vi "Menu-Stop Acq CNV.vi"(11 "Menu in":refnum<k9>) -> ()   [LabVIEW 2016, in "CML UI.lvlib"]
uses:
  CML UI.lvlib
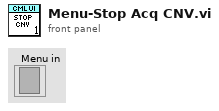
[diagram p1: front panel]
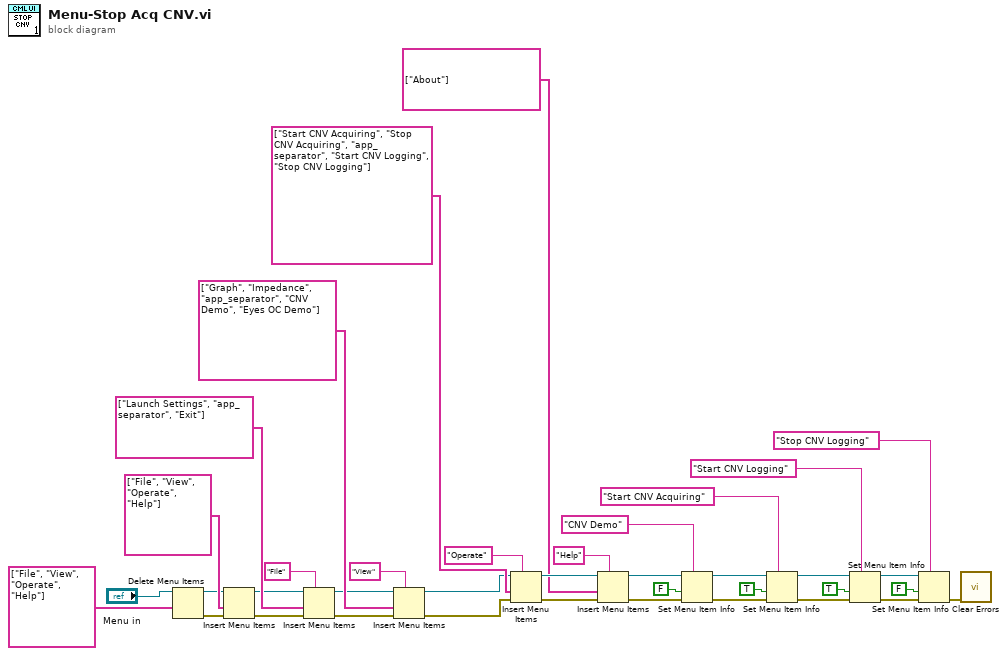
[diagram p0: block diagram]
diagram:
  n1 = Delete Menu Items(7:string[] ["File", "View", "Operate", "Help"] ("L10n_item tags 1"), 9:"Menu in") -> (0:w11:errorcluster, 3:w12:refnum<k9>)  [unwired: 2 in]
  n2 = Insert Menu Items(6:w11, 7:string[] ["File", "View", "Operate", "Help"] ("L10n_item tags 1"), 9:w12) -> (0:w27:errorcluster, 3:w25:refnum<k9>)  [unwired: 3 in, 1 out]
  n3 = Insert Menu Items(5:"File" ("L10n_menu tag"), 6:w27, 7:string[] ["Launch Settings", "app_separator", "Exit"] ("L10n_item tags 2"), 9:w25) -> (0:w32:errorcluster, 3:w31:refnum<k9>)  [unwired: 2 in, 1 out]
  n4 = Insert Menu Items(5:"View" ("L10n_menu tag"), 6:w32, 7:string[] ["Graph", "Impedance", "app_separator", "CNV Demo", "Eyes OC Demo"] ("L10n_item tags 2"), 9:w31) -> (0:w36:errorcluster, 3:w35:refnum<k9>)  [unwired: 2 in, 1 out]
  n5 = Insert Menu Items(5:"Operate" ("L10n_menu tag"), 6:w36, 7:string[] ["Start CNV Acquiring", "Stop CNV Acquiring", "app_separator", "Start CNV Logging", "Stop CNV Logging"] ("L10n_item tags 2"), 9:w35) -> (0:w22:errorcluster, 3:w23:refnum<k9>)  [unwired: 2 in, 1 out]
  n6 = Insert Menu Items(5:"Help" ("L10n_menu tag"), 6:w22, 7:string[] ["About"] ("L10n_item tags 2"), 9:w23) -> (0:w18:errorcluster, 3:w20:refnum<k9>)  [unwired: 2 in, 1 out]
  n7 = Set Menu Item Info(7:"CNV Demo" ("item tag"), 8:w18, 9:FALSE ("enabled"), 11:w20) -> (0:w13:errorcluster, 3:w14:refnum<k9>)  [unwired: 3 in]
  n8 = Set Menu Item Info(7:"Start CNV Acquiring" ("item tag"), 8:w13, 9:TRUE ("enabled"), 11:w14) -> (0:w3:errorcluster, 3:w4:refnum<k9>)  [unwired: 3 in]
  n9 = Set Menu Item Info(7:"Start CNV Logging" ("item tag"), 8:w3, 9:TRUE ("enabled"), 11:w4) -> (0:w10:errorcluster, 3:w9:refnum<k9>)  [unwired: 3 in]
  n10 = Set Menu Item Info(7:"Stop CNV Logging" ("item tag"), 8:w10, 9:FALSE ("enabled"), 11:w9) -> (0:w1:errorcluster)  [unwired: 3 in, 1 out]
  n11 = call <vilib>:"Clear Errors.vi"("error in (no error)"=w1) -> ()  [unwired: 5 in, 2 out]
